vi "WriteRampTable.vi"(8 "error in (no error)":errorcluster, 10 "RampFromFile":dbl[][](array[numeric]) format="%0.3f", 11 "RampProgramModel in":refnum<class "RampProgramModel.lvclass">) -> (0 "error out":errorcluster, 3 "RampProgramModel out":refnum<class "RampProgramModel.lvclass">)   [LabVIEW 2013, in "RampProgramModel.lvclass"]
uses:
  RampProgramModel.lvclass
  RampProgramModel.lvclass/RampProgramModel.ctl
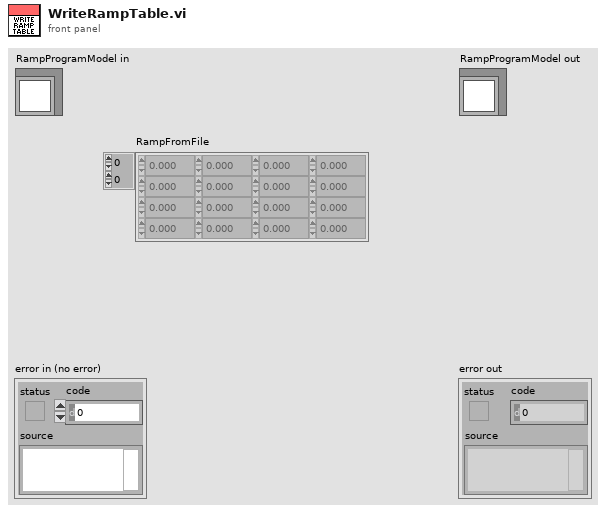
[diagram p1: front panel]
types:
  T1 = cluster{"SP (°C)":dbl, "Cooling rate (°C/min)":dbl, "Dwell Time @ SP (sec)":u32}[]
  T2 = cluster{"SP (°C)":dbl, "Cooling rate (°C/min)":dbl, "Dwell Time @ SP (sec)":u32}
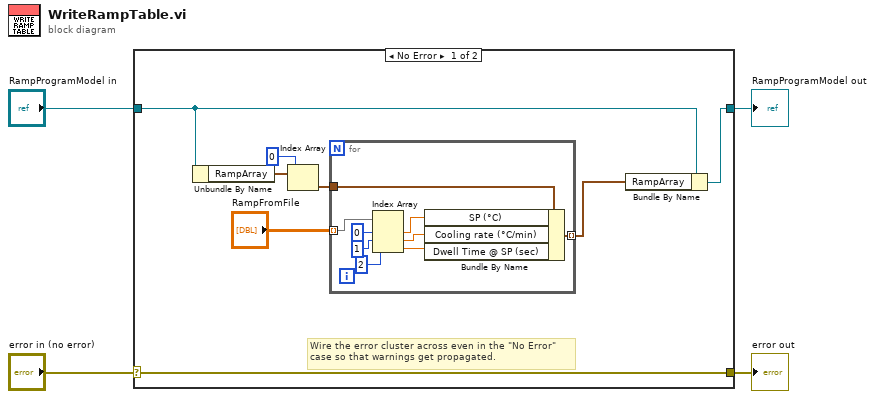
[diagram p0: block diagram]
diagram:
  n1 = case shown="No Error" "error in (no error)" {
    selector: "error in (no error)" -> [w12 w23]
    tunnel: [w12 w23] -> w3
    tunnel: [w11 w22] -> w1
    tunnel: "RampProgramModel in" -> [w9 w22]
    frame No Error {
      # "Wire the error cluster across even in the \"No Error\"\ncase so that warnings get propagated."
      n2 = Unbundle By Name(w9) -> ("RampArray"=w7:T1)
      n3 = Index Array(array=w7, index=0) -> (element=w5:T2)
      n4 = for {
        tunnel: "RampFromFile" -> [w21] mode=indexing
        tunnel: [w17] -> w8 mode=indexing
        tunnel: w5 -> [w13]
        n5 = Index Array(array=w21, index #1=0 ("index"), index #2=1 ("index"), index #3=2 ("index")) -> (element #1=w20:dbl, element #2=w19:dbl, element #3=w18:dbl)
        n6 = Bundle By Name(cluster=w13, "SP (°C)"=w20, "Cooling rate (°C/min)"=w19, "Dwell Time @ SP (sec)"=w18) -> (w17:T2)
      }
      n7 = Bundle By Name(cluster=w9, "RampArray"=w8) -> (w11:refnum<class "RampProgramModel.lvclass">)
    }
    frame Error {
    }
  }
  "error out" <- w3
  "RampProgramModel out" <- w1
